vi "Gasteiler spülen.vi"() -> ()   [LabVIEW 2015, in "Linearisierung v2.lvlib" / "Gasteiler.lvlib"]
uses:
  Gasteiler.lvlib
  AK-Komm Gasteiler/AK Komm Gasteiler.lvlib
  AK-Komm Gasteiler/Aktionen AK Komm.ctl
  Funktionstasten/Funktionstasten.lvlib
  Funktionstasten/Funktionstasten-Aktion.ctl
  Aktionen FGV Gasteiler Daten.ctl
  AK-Komm Gasteiler/Alter Gasteiler/Alter Gasteiler.lvlib
  AK-Komm Gasteiler/Alter Gasteiler/Aktionen AK Komm_ALT.ctl
  Allgemein/allgemeine Sub-VIs.lvlib
  Funktionstasten/Zustaende.ctl
  Visualisierungs Elemente/Button.ctl
  Visualisierungs Elemente/String - Ausgabefeld.ctl
panel:
  out "Gasteiler Status":T1
  in  "NICHT Spülen":T2
  in  "Spülen":T2
  in  "ABBRECHEN":T2
  # "Gasteiler Spülen ?"
  # "Status:"
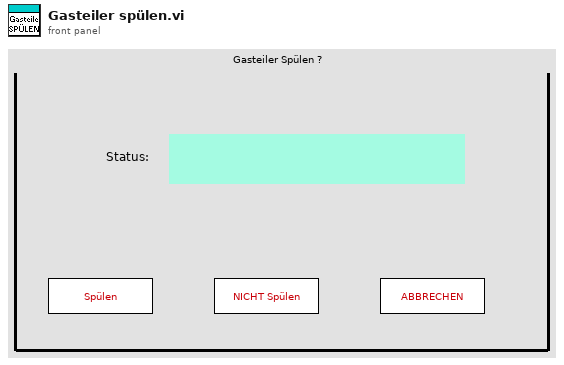
[diagram p1: front panel]
types:
  T1 = typedef "String - Ausgabefeld.ctl" = string
  T2 = typedef "Button.ctl" = bool
  T3 = typedef "Linearisierung v2.lvlib/Gasteiler.lvlib/Aktionen FGV Gasteiler Daten.ctl" = enum16{"lesen", "Gasteiler Daten", "Seriellen Param.", "MB-Endwert", "laden", "speichern", "Anforderung", "TCP", "Aufzeichnung Start"}
  T4 = typedef "Linearisierung v2.lvlib/Gasteiler.lvlib/AK Komm Gasteiler.lvlib/Aktionen AK Komm.ctl" = enum16{"lesen", "initialisieren", "beenden", "Status", "SMAN", "SREM", "STBY", "ASTF", "ASTZ", "SLST", "AGAT", "EGAK", "AGAK", "AKAK", "ADRU", "SKOP", "SVSA", "SVSZ", "SONO", "SAIR", "SNOX", "ANOX", "SSPL", "SRUC", "SLIN", "ALST"}
  T5 = typedef "Linearisierung v2.lvlib/Gasteiler.lvlib/AK Komm Gasteiler.lvlib/Alter Gasteiler.lvlib/Aktionen AK Komm_ALT.ctl" = enum16{"lesen", "initialisieren", "beenden", "SRES", "STBY", "SREM", "SMAN", "SLIN", "SLCH", "SLST", "SSPL", "AGAT", "ALST", "ASTZ", "ASTF", "AGAK", "EGAK"}
  T6 = typedef "Funktionstasten.lvlib/Zustaende.ctl" = enum16{"Standby", "Pause", "Eco", "Messen", "Kalibrieren", "Spülen Filter", "Spülen Leitung", "Umgebungsluft", "0-Gas", "Cal-Gas", "CG zu PNS", "-------------", "Init 1", "Init 2", "Init 3", "Init 4", "Messen vorbereiten", "Messen durchführen", "Exit"}
  T7 = typedef "Funktionstasten.lvlib/Funktionstasten-Aktion.ctl" = enum16{"Initialisieren", "Zustand setzen", "Taste gedrückt", "Fehler speichern", "Lesen", "Manuell", "Remote", "Bitparallel", "Samplepoint", "Zeit Prüfen", "reset Umschalten"}
  T8 = typedef "Neue Linearisierung.lvlib/Gasteiler.lvlib/Gasteiler Type.ctl" = enum16{"LNI Digital", "LNI Analoge", "AVL GDU ", "Horiba GDC"}
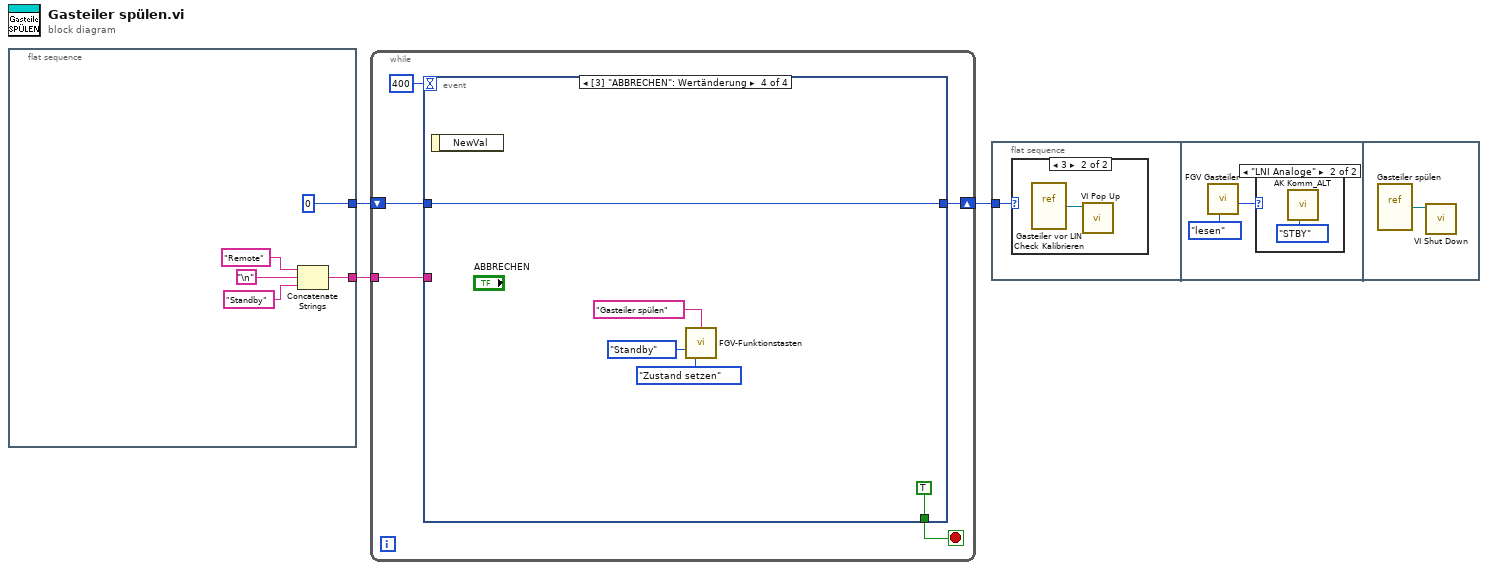
[diagram p0: block diagram]
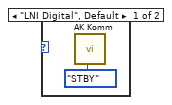
[diagram p3: hidden frame]
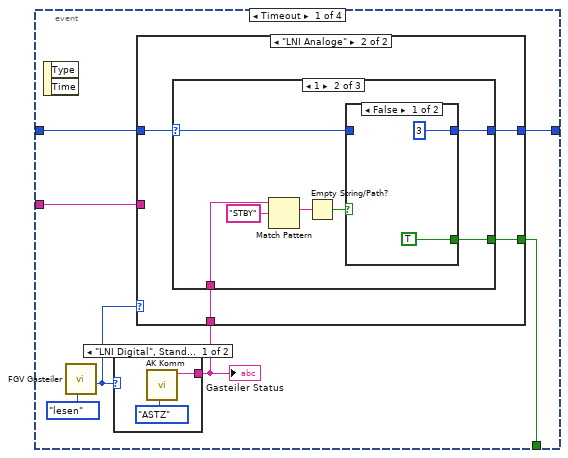
[diagram p4: hidden frame]
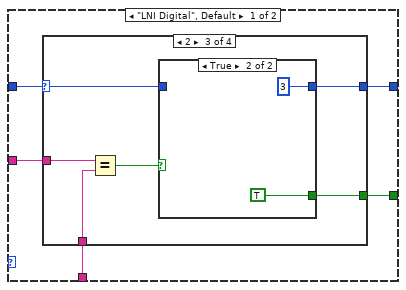
[diagram p5: hidden frame]
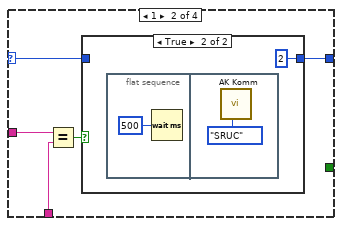
[diagram p7: hidden frame]
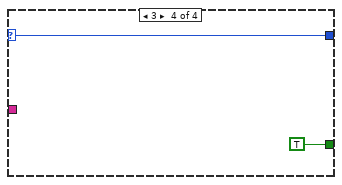
[diagram p10: hidden frame]
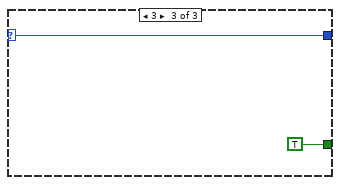
[diagram p13: hidden frame]
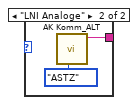
[diagram p14: hidden frame]
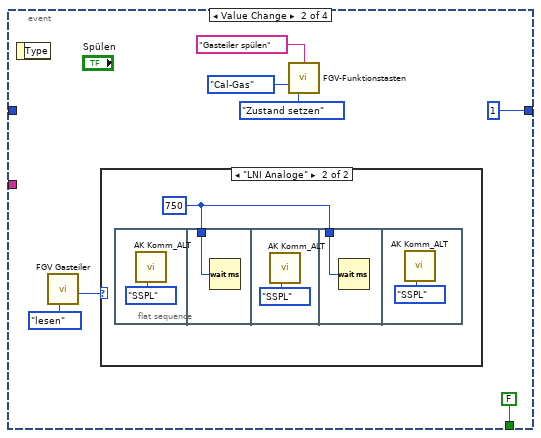
[diagram p15: hidden frame]
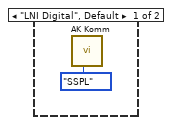
[diagram p16: hidden frame]
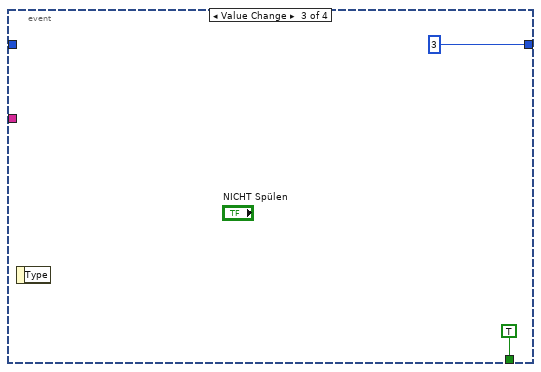
[diagram p17: hidden frame]
diagram:
  n1 = flat-sequence {
    tunnel: [0] -> w3
    tunnel: [w4] -> w1
    frame #0 {
      n2 = Concatenate Strings("Remote", "\n", "Standby") -> (w4:string)
    }
  }
  n3 = while {
    shift-right: [w10] -> w2
    shift-left: w3 -> [w11]
    tunnel: w1 -> [w9]
    stop <- w12 stop-if-true
    n4 = event shown="[3] \"ABBRECHEN\": Wertänderung" {
      selector: _ -> [_ _ _ _]
      dyn-events: _ -> [_ _ _ _]
      timeout: 400 -> [_ _ _ _]
      tunnel: [w18 FALSE ("ABBRECHEN") TRUE ("ABBRECHEN") TRUE ("ABBRECHEN")] -> w12
      tunnel: w11 -> [w20 _ _ w87]
      tunnel: [w19 1 3 w87] -> w10
      tunnel: w9 -> [w16 _ _ _]
      event Timeout {
        n5 = event-data() -> ()  [unwired: 1 in, 2 out]
        n6 = call "FGV Gasteiler.vi"("Aktionen"=Aktionen_FGV_Gasteiler_Daten."lesen") -> ("Gasteiler Type"=w14:T8)  [unwired: 5 in, 5 out]
        n7 = case shown="\"LNI Digital\", Standard" w14 {
          tunnel: [w64 w66] -> w17
          frame "LNI Digital", Default {
            n8 = call "AK Komm.vi"("Aktionen"=Aktionen_AK_Komm."ASTZ") -> ("Status"=w64:string)  [unwired: 5 in, 5 out]
          }
          frame "LNI Analoge" {
            n9 = call "AK Komm_ALT.vi"("Aktionen_ALT"=Aktionen_AK_Komm_ALT."ASTZ") -> ("Status"=w66:string)  [unwired: 6 in, 4 out]
          }
        }
        "Gasteiler Status" <- w17
        n10 = case shown="\"LNI Analoge\"" w14 {
          tunnel: w20 -> [w25 w50]
          tunnel: [w24 w49] -> w19
          tunnel: [w23 w48] -> w18
          tunnel: w17 -> [w22 w47]
          tunnel: w16 -> [w21 _]
          frame "LNI Digital", Default {
            n11 = case shown="2" w25 {
              selector: w25 -> [w26 w30 w40 w46]
              tunnel: [w26 w29 w39 w46] -> w24
              tunnel: [_ _ w38 TRUE] -> w23
              tunnel: w22 -> [_ w28 w37 _]
              tunnel: w21 -> [_ w27 w36 _]
              frame 0, Default {
              }
              frame 1 {
                n12 = Equal?(x=w27, y=w28) -> (x = y?=w31:bool)
                n13 = case shown="True" w31 {
                  tunnel: w30 -> [w32 _]
                  tunnel: [w32 2] -> w29
                  frame False {
                  }
                  frame True {
                    n14 = flat-sequence {
                      frame #0 {
                        n15 = Wait (ms)(milliseconds to wait=u32 500 ("Zu wartende ms")) -> ()  [unwired: 1 out]
                      }
                      frame #1 {
                        n16 = call "AK Komm.vi"("Aktionen"=Aktionen_AK_Komm."SRUC") -> ()  [unwired: 5 in, 6 out]
                      }
                    }
                  }
                }
              }
              frame 2 {
                n17 = Equal?(x=w36, y=w37) -> (x = y?=w41:bool)
                n18 = case shown="True" w41 {
                  tunnel: w40 -> [w42 _]
                  tunnel: [w42 3] -> w39
                  tunnel: [_ TRUE] -> w38
                  frame False {
                  }
                  frame True {
                  }
                }
              }
              frame 3 {
              }
            }
          }
          frame "LNI Analoge" {
            n19 = case shown="1" w50 {
              selector: w50 -> [w51 w58 w63]
              tunnel: [w51 w57 w63] -> w49
              tunnel: [_ w52 TRUE] -> w48
              tunnel: w47 -> [_ w54 _]
              frame 0, Default {
              }
              frame 1 {
                n20 = Match Pattern(string=w54, regular expression="STBY" ("Regulärer Ausdruck")) -> (match substring=w55:string)  [unwired: 1 in, 3 out]
                n21 = Empty String/Path?(string/path=w55) -> (empty?=w53:bool)
                n22 = case shown="False" w53 {
                  tunnel: w58 -> [_ w61]
                  tunnel: [3 w61] -> w57
                  tunnel: [TRUE _] -> w52
                  frame False {
                  }
                  frame True {
                  }
                }
              }
              frame 3 {
              }
            }
          }
        }
      }
      event Value Change {
        n23 = event-data() -> ()  [unwired: 1 in, 1 out]
        n24 = call "FGV Gasteiler.vi"("Aktionen"=Aktionen_FGV_Gasteiler_Daten."lesen") -> ("Gasteiler Type"=w72:T8)  [unwired: 5 in, 5 out]
        n25 = case shown="\"LNI Analoge\"" w72 {
          frame "LNI Digital", Default {
            n26 = call "AK Komm.vi"("Aktionen"=Aktionen_AK_Komm."SSPL") -> ()  [unwired: 5 in, 6 out]
          }
          frame "LNI Analoge" {
            w76 = u32 750 ("Zu wartende ms")
            n27 = flat-sequence {
              tunnel: w76 -> [w78]
              tunnel: w76 -> [w80]
              frame #0 {
                n28 = call "AK Komm_ALT.vi"("Aktionen_ALT"=Aktionen_AK_Komm_ALT."SSPL") -> ()  [unwired: 6 in, 5 out]
              }
              frame #1 {
                n29 = Wait (ms)(milliseconds to wait=w78) -> ()  [unwired: 1 out]
              }
              frame #2 {
                n30 = call "AK Komm_ALT.vi"("Aktionen_ALT"=Aktionen_AK_Komm_ALT."SSPL") -> ()  [unwired: 6 in, 5 out]
              }
              frame #3 {
                n31 = Wait (ms)(milliseconds to wait=w80) -> ()  [unwired: 1 out]
              }
              frame #4 {
                n32 = call "AK Komm_ALT.vi"("Aktionen_ALT"=Aktionen_AK_Komm_ALT."SSPL") -> ()  [unwired: 6 in, 5 out]
              }
            }
          }
        }
        n33 = call "FGV-Funktionstasten.vi"("Herkunft"="Gasteiler spülen", "Zustand"=Zustaende."Cal-Gas", "Aktion"=Funktionstasten-Aktion."Zustand setzen") -> ()  [unwired: 7 in, 6 out]
      }
      event Value Change {
        n34 = event-data() -> ()  [unwired: 1 in, 1 out]
      }
      event Value Change {
        n35 = event-data() -> ()  [unwired: 1 in, 1 out]
        n36 = call "FGV-Funktionstasten.vi"("Herkunft"="Gasteiler spülen", "Zustand"=Zustaende."Standby", "Aktion"=Funktionstasten-Aktion."Zustand setzen") -> ()  [unwired: 7 in, 6 out]
      }
    }
  }
  n37 = flat-sequence {
    tunnel: w2 -> [w89]
    frame #0 {
      n38 = case shown="3" w89 {
        frame 0, Default {
        }
        frame 3 {
          n39 = vi-ref "Gasteiler vor LIN Check Kalibrieren.vi"() -> (w90:refnum<vi>)
          n40 = call "VI Pop Up.vi"("VI Referenz"=w90) -> ()  [unwired: 11 in]
        }
      }
    }
    frame #1 {
      n41 = call "FGV Gasteiler.vi"("Aktionen"=Aktionen_FGV_Gasteiler_Daten."lesen") -> ("Gasteiler Type"=w91:T8)  [unwired: 5 in, 5 out]
      n42 = case shown="\"LNI Analoge\"" w91 {
        frame "LNI Digital", Default {
          n43 = call "AK Komm.vi"("Aktionen"=Aktionen_AK_Komm."STBY") -> ()  [unwired: 5 in, 6 out]
        }
        frame "LNI Analoge" {
          n44 = call "AK Komm_ALT.vi"("Aktionen_ALT"=Aktionen_AK_Komm_ALT."STBY") -> ()  [unwired: 6 in, 5 out]
        }
      }
    }
    frame #2 {
      n45 = vi-ref "Gasteiler spülen.vi"() -> (w95:refnum<vi>)
      n46 = call "VI Shut Down.vi"("VI Referenz"=w95) -> ()  [unwired: 11 in]
    }
  }
